vi "ColorMixture.vi"(1 "Concentration1":dbl min=0.0 max=1.0, 2 "Reflectance spectrum 2":dbl[](array[numeric]), 3 "Reflectance spectrum":dbl[](array[numeric])) -> (0 "Mixtured colors":dbl[](array[numeric]))   [LabVIEW 2013]
uses:
  <vilib>/Utility/file.llb/Write To Spreadsheet File (DBL).vi
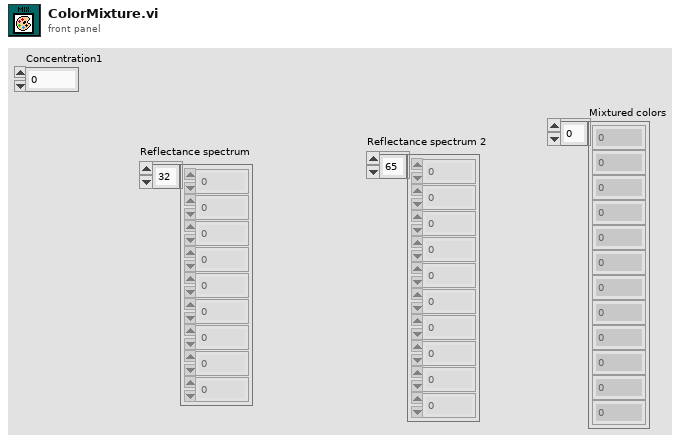
[diagram p1: front panel]
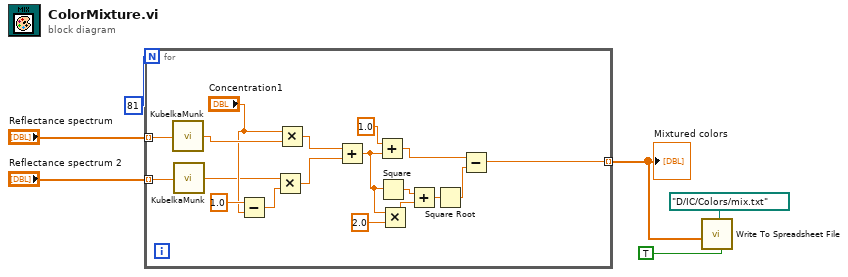
[diagram p0: block diagram]
diagram:
  n1 = for {
    N: 81 -> [_]
    tunnel: "Reflectance spectrum" -> [w24] mode=indexing
    tunnel: "Reflectance spectrum 2" -> [w23] mode=indexing
    tunnel: [w14] -> w3 mode=indexing
    n2 = call "KubelkaMunk.vi"("Reflectance"=w24) -> ("K/S"=w13:dbl)
    n3 = call "KubelkaMunk.vi"("Reflectance"=w23) -> ("K/S"=w9:dbl)
    n4 = Subtract(x=1.0, y="Concentration1") -> (x-y=w10:dbl)
    n5 = Multiply(x=w9, y=w10) -> (x*y=w7:dbl)
    n6 = Multiply(x="Concentration1", y=w13) -> (x*y=w8:dbl)
    n7 = Add(x=w8, y=w7) -> (x+y=w18:dbl)
    n8 = Add(x=1.0, y=w18) -> (x+y=w21:dbl)
    n9 = Square(x=w18) -> (x^2=w20:dbl)
    n10 = Multiply(x=w18, y=2.0) -> (x*y=w19:dbl)
    n11 = Add(x=w20, y=w19) -> (x+y=w16:dbl)
    n12 = Square Root(x=w16) -> (sqrt(x)=w15:dbl)
    n13 = Subtract(x=w21, y=w15) -> (x-y=w14:dbl)
  }
  "Mixtured colors" <- w3
  n14 = call-poly <vilib>:"Write To Spreadsheet File.vi"("transpose? (no:F)"=TRUE, "1D data"=w3, "file path (dialog if empty)"=path "D:/IC/Colors/mix.txt") -> ()  [unwired: 5 in, 1 out]
